vi "Enable Tare Offset.vi"(6 "Enable Tare (Off)":bool, 7 "Channel (0: Channel A)":u16(ring) items=["Channel A", "Channel B"], 8 "error in (no error)":errorcluster, 9 "Manual Tare Offset":dbl, 10 "Tare Source (0: Auto)":enum16{"Auto", "Manual"}(ring)=enum."Manual", 11 "BH Druck PACE Series in":refnum<class "BH Druck PACE Series.lvclass">) -> (0 "error out":errorcluster, 2 "Tare Offset":dbl, 3 "BH Druck PACE Series out":refnum<class "BH Druck PACE Series.lvclass">)   [LabVIEW 2022 SP3, in "BH Druck PACE Series.lvclass"]
uses:
  BH Druck PACE Series.lvclass
  BH Druck PACE Series.lvclass/BH Druck PACE Series.ctl
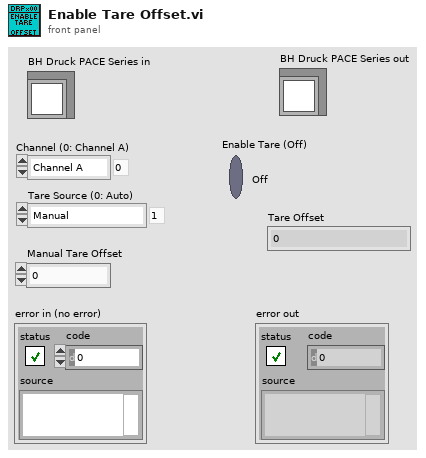
[diagram p1: front panel]
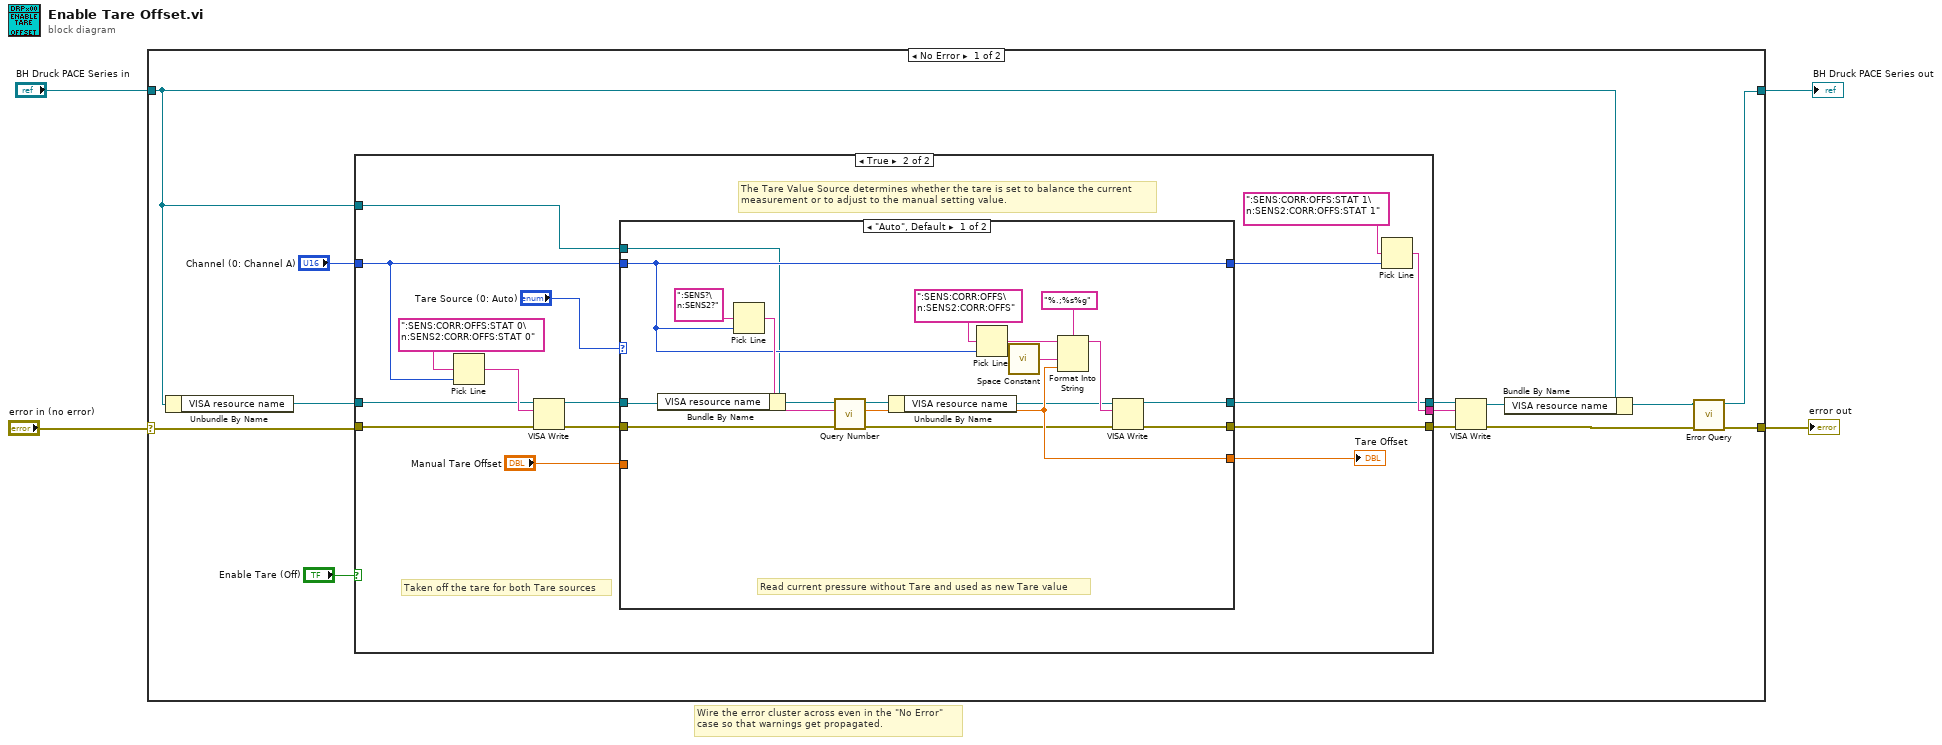
[diagram p0: block diagram]
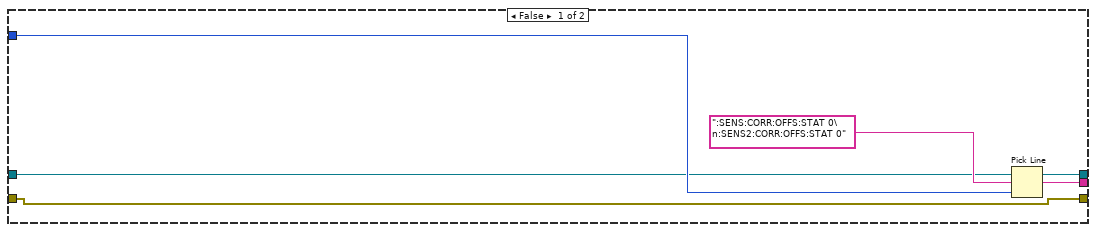
[diagram p2: hidden frame]
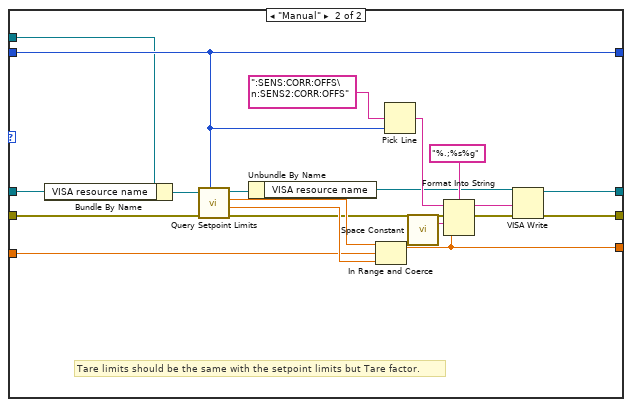
[diagram p3: hidden frame]
diagram:
  # "Wire the error cluster across even in the \"No Error\"\ncase so that warnings get propagated."
  n1 = case shown="No Error" "error in (no error)" {
    selector: "error in (no error)" -> [w12 w78]
    tunnel: [w7 w78] -> w3
    tunnel: [w5 w77] -> w1
    tunnel: "BH Druck PACE Series in" -> [w10 w77]
    frame No Error {
      n2 = Unbundle By Name(w10) -> ("VISA resource name"=w11:refnum<visa-resource-name>)
      n3 = case shown="True" "Enable Tare (Off)" {
        tunnel: "Channel (0: Channel A)" -> [w21 w25]
        tunnel: [w20 w34] -> w15
        tunnel: [w19 w33] -> w14
        tunnel: [w18 w32] -> w13
        tunnel: w11 -> [w19 w29]
        tunnel: w12 -> [w18 w27]
        tunnel: w10 -> [_ w23]
        frame False {
          n4 = Pick Line(multi-line string=":SENS:CORR:OFFS:STAT 0\n:SENS2:CORR:OFFS:STAT 0", line index=w21) -> (output string=w20:string)  [unwired: 1 in]
        }
        frame True {
          # "Taken off the tare for both Tare sources"
          # "The Tare Value Source determines whether the tare is set to balance the current\nmeasurement or to adjust to the manual setting value."
          n5 = Pick Line(multi-line string=":SENS:CORR:OFFS:STAT 0\n:SENS2:CORR:OFFS:STAT 0", line index=w25) -> (output string=w30:string)  [unwired: 1 in]
          n6 = VISA Write(VISA resource name=w29, write buffer=w30, error in (no error)=w27) -> (VISA resource name out=w28:refnum<visa-resource-name>, error out=w26:errorcluster)  [unwired: 1 out]
          n7 = case shown="\"Auto\", Default" "Tare Source (0: Auto)" {
            tunnel: "Manual Tare Offset" -> [_ w69]
            tunnel: w28 -> [w42 w60]
            tunnel: w26 -> [w50 w64]
            tunnel: w25 -> [w48 w67]
            tunnel: [w49 w63] -> w24
            tunnel: [w48 w67] -> w35
            tunnel: [w47 w66] -> w33
            tunnel: [w46 w65] -> w32
            tunnel: w23 -> [w43 w61]
            frame "Auto", Default {
              # "Read current pressure without Tare and used as new Tare value"
              n8 = Bundle By Name(cluster=w43, "VISA resource name"=w42) -> (w41:refnum<class "BH Druck PACE Series.lvclass">)
              n9 = Pick Line(multi-line string=":SENS?\n:SENS2?", line index=w48) -> (output string=w54:string)  [unwired: 1 in]
              n10 = call-dynamic "Query Number.vi"("error in (no error)"=w50, "Query String"=w54, "BH Druck PACE Series in"=w41) -> ("error out"=w45:errorcluster, "Numeric Result"=w49:dbl, "BH Druck PACE Series out"=w40:refnum<class "BH Druck PACE Series.lvclass">)  [unwired: 6 in]
              n11 = Unbundle By Name(w40) -> ("VISA resource name"=w39:refnum<visa-resource-name>)
              n12 = Pick Line(multi-line string=":SENS:CORR:OFFS\n:SENS2:CORR:OFFS", line index=w48) -> (output string=w56:string)  [unwired: 1 in]
              n13 = call <vilib>:"Space Constant.vi"() -> ("String"=w51:string)
              n14 = Format Into String(format string="%.;%s%g", initial string=w56, w51, w49) -> (resulting string=w55:string)  [unwired: 1 in, 1 out]
              n15 = VISA Write(VISA resource name=w39, write buffer=w55, error in (no error)=w45) -> (VISA resource name out=w47:refnum<visa-resource-name>, error out=w46:errorcluster)  [unwired: 1 out]
            }
            frame "Manual" {
              # "Tare limits should be the same with the setpoint limits but Tare factor."
              n16 = Bundle By Name(cluster=w61, "VISA resource name"=w60) -> (w59:refnum<class "BH Druck PACE Series.lvclass">)
              n17 = call-dynamic "Query Setpoint Limits.vi"("Channel (0: Channel A)"=w67, "error in (no error)"=w64, "BH Druck PACE Series in"=w59) -> ("error out"=w68:errorcluster, "Lower Setpoint Limit"=w70:dbl, "Upper Setpoint Limit"=w71:dbl, "BH Druck PACE Series out"=w58:refnum<class "BH Druck PACE Series.lvclass">)  [unwired: 5 in]
              n18 = Unbundle By Name(w58) -> ("VISA resource name"=w57:refnum<visa-resource-name>)
              n19 = In Range and Coerce(upper limit=w71, x=w69, lower limit=w70) -> (coerced(x)=w63:dbl)  [unwired: 1 out]
              n20 = Pick Line(multi-line string=":SENS:CORR:OFFS\n:SENS2:CORR:OFFS", line index=w67) -> (output string=w76:string)  [unwired: 1 in]
              n21 = call <vilib>:"Space Constant.vi"() -> ("String"=w74:string)
              n22 = Format Into String(format string="%.;%s%g", initial string=w76, error in=w68, w74, w63) -> (resulting string=w75:string, error out=w72:errorcluster)
              n23 = VISA Write(VISA resource name=w57, write buffer=w75, error in (no error)=w72) -> (VISA resource name out=w66:refnum<visa-resource-name>, error out=w65:errorcluster)  [unwired: 1 out]
            }
          }
          "Tare Offset" <- w24
          n24 = Pick Line(multi-line string=":SENS:CORR:OFFS:STAT 1\n:SENS2:CORR:OFFS:STAT 1", line index=w35) -> (output string=w34:string)  [unwired: 1 in]
        }
      }
      n25 = VISA Write(VISA resource name=w14, write buffer=w15, error in (no error)=w13) -> (VISA resource name out=w9:refnum<visa-resource-name>, error out=w8:errorcluster)  [unwired: 1 out]
      n26 = Bundle By Name(cluster=w10, "VISA resource name"=w9) -> (w6:refnum<class "BH Druck PACE Series.lvclass">)
      n27 = call-dynamic "Error Query.vi"("error in (no error)"=w8, "BH Druck PACE Series in"=w6) -> ("error out"=w7:errorcluster, "BH Druck PACE Series out"=w5:refnum<class "BH Druck PACE Series.lvclass">)  [unwired: 8 in]
    }
    frame Error {
    }
  }
  "error out" <- w3
  "BH Druck PACE Series out" <- w1
